vi "get tilt state mks.vi"(8 "error in (no error)":errorcluster, 11 "index":i32) -> (0 "error out":errorcluster, 1 "dz out":dbl, 2 "dy out":dbl, 3 "dx out":dbl)   [LabVIEW 2010, in "libfreenect.lvlib"]
doc: "EXPORT void freenect_lv_get_tilt_state_mks(double *dx, double *dy, double *dz, int index);"
uses:
  libfreenect.lvlib
  freenect_lv.dll
panel:
  in  "dz":dbl
  in  "dy":dbl
  in  "dx":dbl
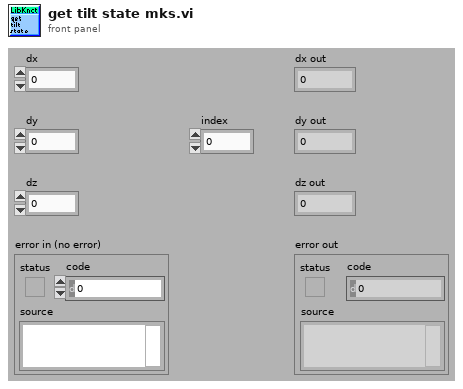
[diagram p1: front panel]
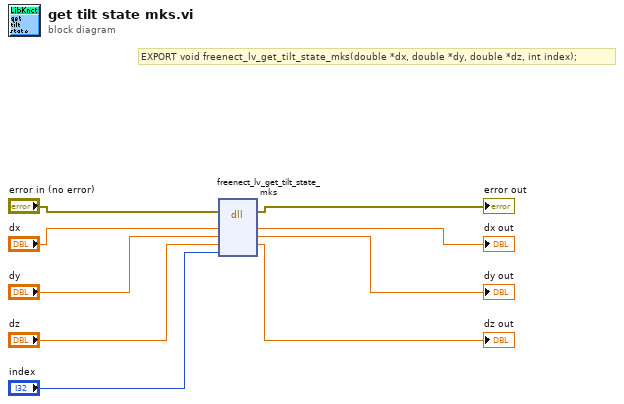
[diagram p0: block diagram]
diagram:
  # "EXPORT void freenect_lv_get_tilt_state_mks(double *dx, double *dy, double *dz, int index);"
  n1 = dll-call lib="C:/Users/anfedres/Desktop/Tesis/G-BAR/wrappers/labview/lvlib - copia/freenect_lv.*" fn="freenect_lv_get_tilt_state_mks"(error in="error in (no error)", "dx"="dx", "dy"="dy", "dz"="dz", "index"="index") -> (error out=→"error out":errorcluster, "dx"=→"dx out":dbl, "dy"=→"dy out":dbl, "dz"=→"dz out":dbl)  [unwired: 3 in, 2 out]
